vi "Sets the FAIL mode for MANU.vi"(5 "Enable to Query the FAIL mode":bool, 7 "Enable to Setup the FAIL mode":bool, 8 "error in":errorcluster, 10 "FAIL mode Setting":u8(ring) items=["STOP", "CONT", "HOLD"], 11 "VISA resource name":refnum<visa-resource-name>) -> (0 "error out":errorcluster, 2 "Return the FAIL mode Setting":string, 3 "VISA resource name out":refnum<visa-resource-name>)   [LabVIEW 2011, in "GPT-9000.lvlib"]
uses:
  <instrlib>/GPT-9000/GPT-9000.lvlib
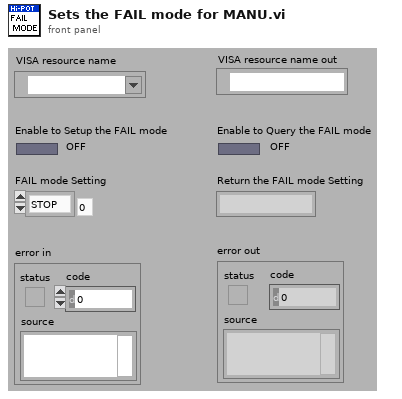
[diagram p1: front panel]
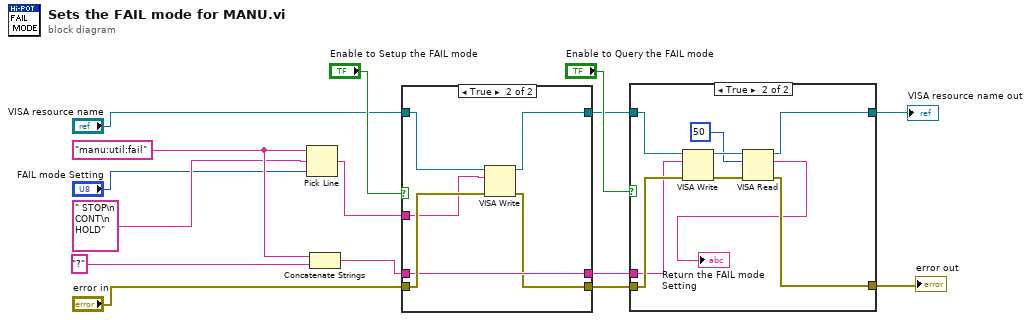
[diagram p0: block diagram]
diagram:
  w4 = "manu:util:fail"
  n1 = Pick Line(string ("")=w4, multi-line string=" STOP\n CONT\n HOLD", line index="FAIL mode Setting") -> (output string=w1:string)
  n2 = Concatenate Strings(w4, "?") -> (w13:string)
  n3 = case shown="True" "Enable to Setup the FAIL mode" {
    tunnel: w1 -> [_ w22]
    tunnel: w13 -> [w16 w21]
    tunnel: "VISA resource name" -> [w18 w24]
    tunnel: "error in" -> [w17 w23]
    tunnel: [w18 w20] -> w9
    tunnel: [w17 w19] -> w8
    tunnel: [w16 w21] -> w7
    frame False {
    }
    frame True {
      n4 = VISA Write(VISA resource name=w24, write buffer=w22, error in (no error)=w23) -> (VISA resource name out=w20:refnum<visa-resource-name>, error out=w19:errorcluster)  [unwired: 1 out]
    }
  }
  n5 = case shown="True" "Enable to Query the FAIL mode" {
    tunnel: w9 -> [w26 w32]
    tunnel: w8 -> [w25 w31]
    tunnel: w7 -> [_ w30]
    tunnel: [w26 w29] -> w6
    tunnel: [w25 w28] -> w5
    frame False {
    }
    frame True {
      n6 = VISA Write(VISA resource name=w32, write buffer=w30, error in (no error)=w31) -> (VISA resource name out=w34:refnum<visa-resource-name>, error out=w35:errorcluster)  [unwired: 1 out]
      n7 = VISA Read(VISA resource name=w34, byte count=u32 50, error in (no error)=w35) -> (VISA resource name out=w29:refnum<visa-resource-name>, read buffer=→"Return the FAIL mode Setting":string, error out=w28:errorcluster)  [unwired: 1 out]
    }
  }
  "VISA resource name out" <- w6
  "error out" <- w5
